vi "Main_Fun_Enqueue.vi"(7 "Priority Message (F)":bool, 8 "Error in":errorcluster, 9 "Message Data":variant, 10 "Queue Action":T1=enum."動作-系統初始化", 11 "Message Queue":refnum<queue>) -> (0 "Error Out":errorcluster, 3 "Message Queue Out":refnum<queue>)   [LabVIEW 2015]
uses:
  Control_Main_QData.ctl
  Control_Main_Queue Action.ctl
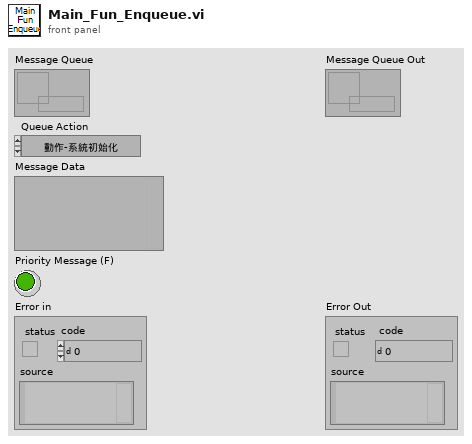
[diagram p1: front panel]
types:
  T1 = typedef "Control_Main_Queue Action.ctl" = enum16{"動作-使用者登入", "動作-系統初始化", "動作-開始", "動作-系統管理選單", "動作-資料管理", "動作-登出/離開", "動作-關於本系統", "1.0 帳號管理", "    1.1 登入", "    1.2 確認狀態", "    1.3 更新介面", "    1.4 帳號管理", "    1.5 登出", "2.0 每日點檢", "10.0 系統", "    10.1 系統-關機", "    10.2 系統-等待", "    10.3 系統-回到作業系統"}
  T2 = typedef "Control_Main_QData.ctl" = cluster{"Queue Action":T1, "Queue Data":variant}
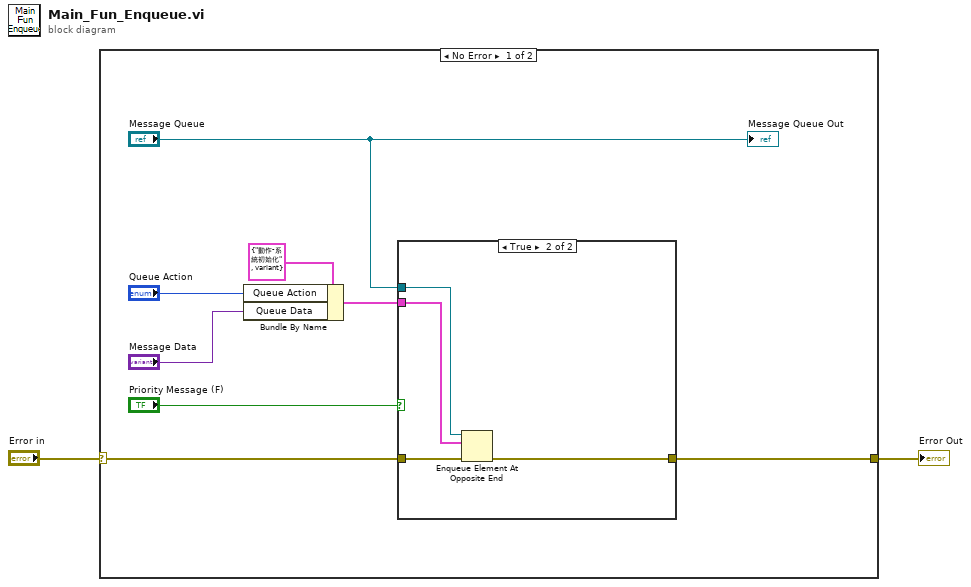
[diagram p0: block diagram]
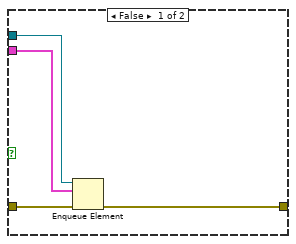
[diagram p2: hidden frame]
diagram:
  n1 = case shown="No Error" "Error in" {
    selector: "Error in" -> [w3 w19]
    tunnel: [w7 w19] -> w2
    frame No Error {
      n2 = Bundle By Name(cluster=T2 {"Queue Action"=enum."動作-系統初始化", "Queue Data"=variant} ("Queue Data"), "Queue Action"="Queue Action", "Queue Data"="Message Data") -> (w10:T2)
      n3 = case shown="True" "Priority Message (F)" {
        tunnel: w3 -> [w14 w18]
        tunnel: [w13 w17] -> w7
        tunnel: "Message Queue" -> [w12 w16]
        tunnel: w10 -> [w11 w15]
        frame False {
          n4 = Enqueue Element(queue=w12, element=w11, error in (no error)=w14) -> (error out=w13:errorcluster)  [unwired: 1 in, 2 out]
        }
        frame True {
          n5 = Enqueue Element At Opposite End(queue=w16, element=w15, error in (no error)=w18) -> (error out=w17:errorcluster)  [unwired: 1 in, 2 out]
        }
      }
      "Message Queue Out" <- "Message Queue"
    }
    frame Error {
    }
  }
  "Error Out" <- w2
